vi "Save Test Data.vi"(8 "error in (no error)":errorcluster, 10 "Test Data":string[](array[string]), 11 "MySQL in":refnum<class "MySQL.lvclass">) -> (0 "error out":errorcluster, 3 "MySQL out":refnum<class "MySQL.lvclass">)   [LabVIEW 2021, in "Database.lvlib" / "MySQL.lvclass"]
uses:
  MySQL.lvclass
  User Interface/Test Info.ctl
  MySQL.lvclass/MySQL.ctl
  <vilib>/addons/database/NI_Database_API.lvlib
  User Interface/User Interface.lvlib
panel:
  in  "Test info":T1
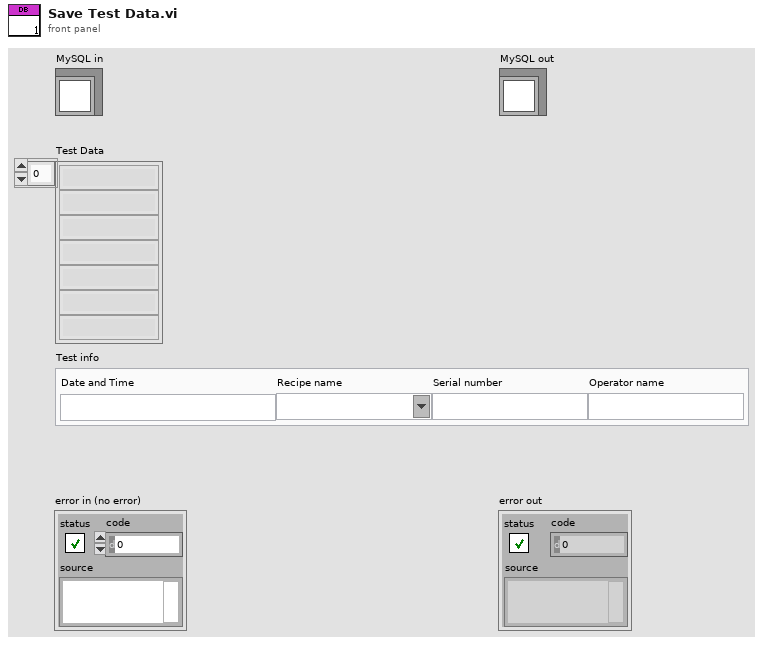
[diagram p1: front panel]
types:
  T1 = typedef "User Interface.lvlib/Test Info.ctl" = cluster{"Date and Time":string, "Recipe name":string, "Serial number":string, "Operator name":string}
  T2 = typedef "Database.lvlib/DB.lvclass/Table_info.ctl" = cluster{"Authentication":string, "Instr_Configuration":string, "Recipe":string, "Test_data":string}
  T3 = typedef "NI_Database_API.lvlib/Conn ObjectReference.ctl" = refnum<k1>
  T4 = cluster{"[0]":string, "[1]":string, "[2]":string, "[3]":string, "[4]":string, "[5]":string, "[6]":string, "[7]":string, "[8]":string, "[9]":string, "[10]":string, "[11]":string, "[12]":string, "[13]":string}
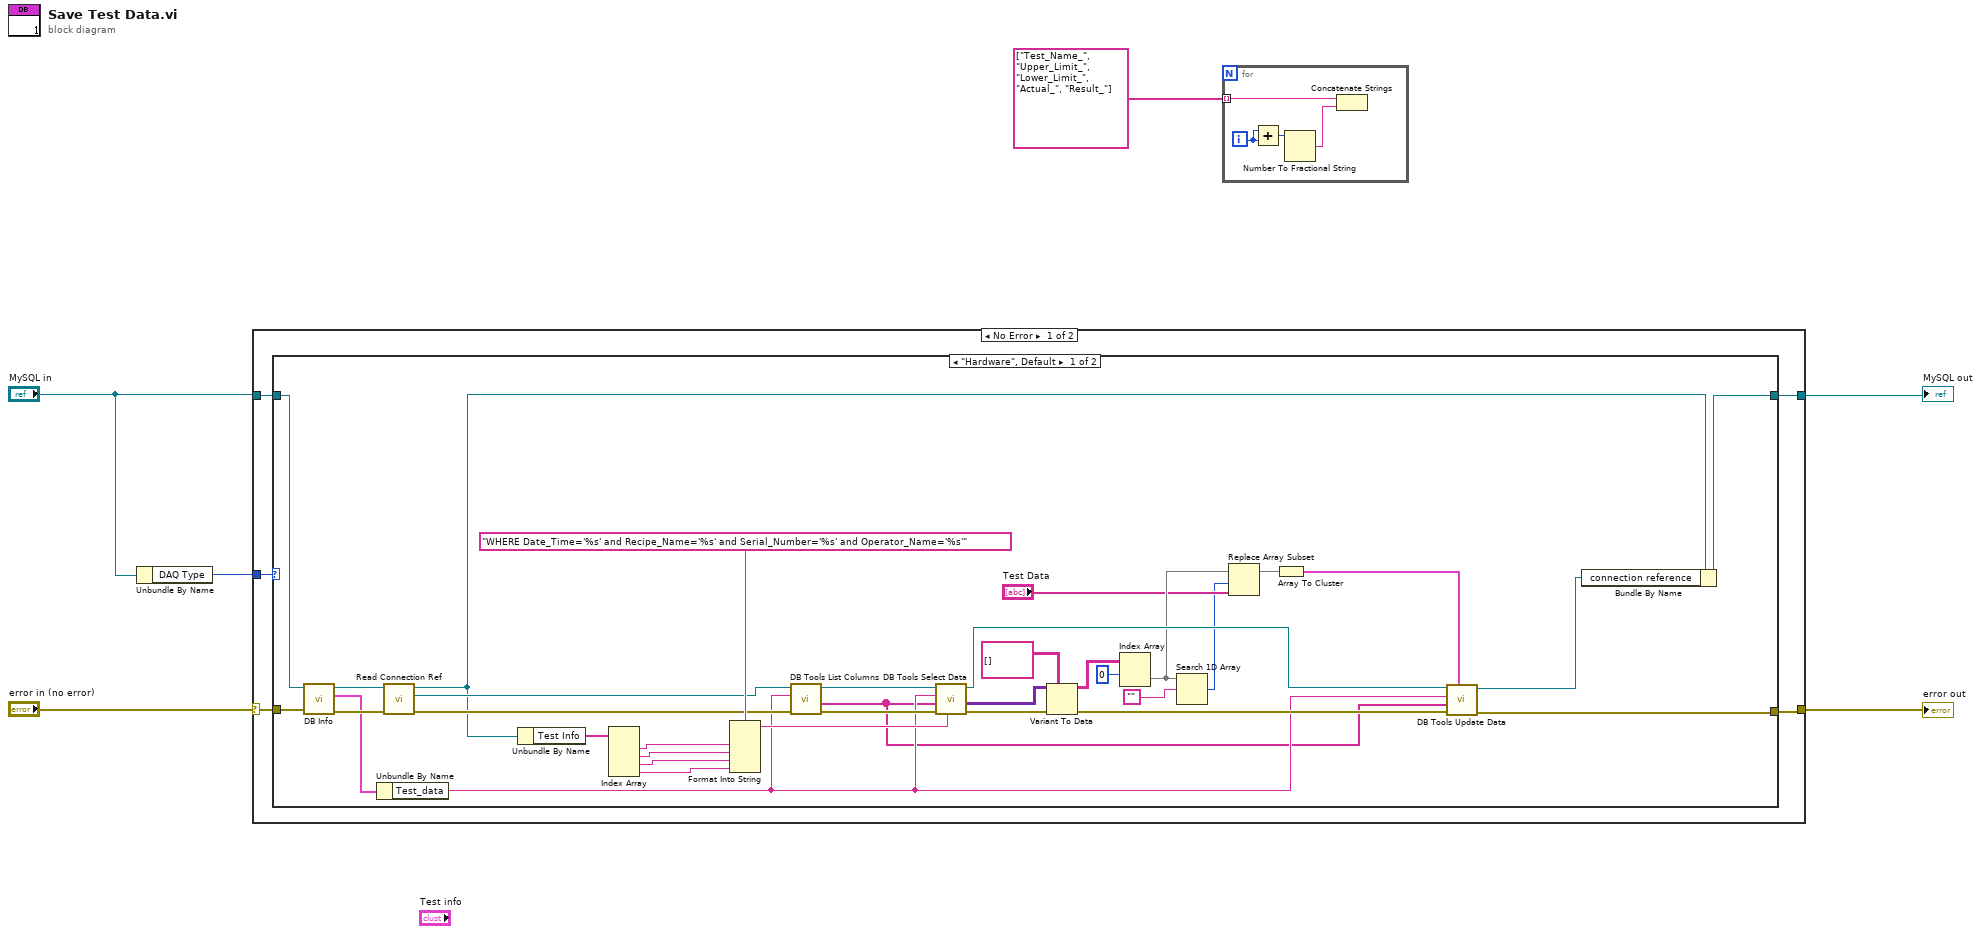
[diagram p0: block diagram]
diagram:
  n1 = Unbundle By Name("MySQL in") -> ("DAQ Type"=w6:enum16{"Hardware", "Simulation"})
  n2 = case shown="No Error" "error in (no error)" {
    selector: "error in (no error)" -> [w11 w50]
    tunnel: "MySQL in" -> [w10 w49]
    tunnel: [w8 w49] -> w2
    tunnel: [w9 w50] -> w3
    tunnel: w6 -> [w7 _]
    frame No Error {
      n3 = case shown="\"Hardware\", Default" w7 {
        tunnel: w11 -> [w46 w47]
        tunnel: w10 -> [w41 w48]
        tunnel: [w19 w47] -> w9
        tunnel: [w43 w48] -> w8
        frame "Hardware", Default {
          n4 = call-dynamic "DB Info.vi"("error in (no error)"=w46, "MySQL in"=w41) -> ("error out"=w45:errorcluster, "Table_info"=w42:T2, "MySQL out"=w44:refnum<class "MySQL.lvclass">)  [unwired: 6 in, 1 out]
          n5 = Unbundle By Name(w42) -> ("Test_data"=w23:string)
          n6 = call-dynamic "Read Connection Ref.vi"("error in (no error)"=w45, "MySQL in"=w44) -> ("error out"=w38:errorcluster, "connection reference"=w37:T3, "MySQL out"=w35:refnum<class "MySQL.lvclass">)  [unwired: 7 in]
          n7 = Unbundle By Name(w35) -> ("Test Info"=w34:string[])
          n8 = Index Array(array=w34) -> (element #1=w33:string, element #2=w32:string, element #3=w31:string, element #4=w30:string)  [unwired: 4 in]
          n9 = Format Into String(format string="WHERE Date_Time='%s' and Recipe_Name='%s' and Serial_Number='%s' and Operator_Name='%s'" ("condition"), w33, w32, w31, w30) -> (resulting string=w39:string)  [unwired: 2 in, 1 out]
          n10 = call <vilib>:"DB Tools List Columns.vi"("error in (no error)"=w38, "table"=w23, "connection reference"=w37) -> ("error out"=w26:errorcluster, "columns"=w22:string[], "connection reference out"=w36:T3)  [unwired: 1 in, 1 out]
          n11 = call <vilib>:"DB Tools Select Data.vi"("condition"=w39, "error in (no error)"=w26, "columns"=w22, "table"=w23, "connection reference"=w36) -> ("error out"=w29:errorcluster, "data"=w28:variant[][], "connection reference out"=w25:T3)  [unwired: 1 in]
          n12 = Variant To Data(error in=w29, type=string[][] [], Variant=w28) -> (data=w18:string[][], error out=w24:errorcluster)
          n13 = Index Array(array=w18, index (row)=0 ("disabled index (col)")) -> (element=w16:string[])  [unwired: 1 in]
          n14 = Search 1D Array(1D array=w16, element="") -> (index of element=w14:i32)  [unwired: 1 in]
          n15 = Replace Array Subset(array=w16, new element="Test Data", index=w14) -> (w13:string[])
          n16 = Array To Cluster(array=w13) -> (cluster=w21:T4)
          n17 = call <vilib>:"DB Tools Update Data.vi"("data"=w21, "error in (no error)"=w24, "columns"=w22, "table"=w23, "connection reference"=w25) -> ("error out"=w19:errorcluster, "connection reference out"=w20:T3)  [unwired: 5 in]
          n18 = Bundle By Name(cluster=w35, "connection reference"=w20) -> (w43:refnum<class "MySQL.lvclass">)
        }
        frame "Simulation" {
        }
      }
    }
    frame Error {
    }
  }
  "error out" <- w3
  "MySQL out" <- w2
  n19 = for {
    tunnel: string[] ["Test_Name_", "Upper_Limit_", "Lower_Limit_", "Actual_", "Result_"] -> [w53] mode=indexing
    i -> [w51]
    n20 = Add(x=w51, y=w51) -> (x+y=w52:i32)
    n21 = Number To Fractional String(number=w52) -> (F-format string=w54:string)  [unwired: 3 in]
    n22 = Concatenate Strings(w53, w54) -> ()  [unwired: 1 out]
  }
